vi "pixelfly_init.vi"(3 "error in (no error)":errorcluster, 4 "PixelFly Controls":T1={"Acquitsition Settings"={"Buffer number"=1, "Size (Bytes)"=150, "initialized array"=array2048x1280[2621440 elements], "X Bin"=1, "Y Bin"=0, "Board Handle"=0, "Picture parameters"={"ccdxsize"=0, "ccdy"=0, "pictx"=0, "picty"=0, "bitspixel"=12}, "Buffer Out"=[]}, "Initialization"={"Exposure mode"=1, "exp time"=150, "exp level"=1, "gain"=0, "boardid in"=0, "offset"=0, "V bin"=0, "H bin"=0, "trigger"=TRUE, "Bit depth"=0}} {"Initialization"."Bit depth" items=["8", "12"]; "Initialization"."H bin" items=["1", "2"]; "Initialization"."V bin" items=["1", "2"]; "Initialization"."boardid in" min=0 max=3 step=1; "Initialization"."gain" items=["Low (X1)", "High (X2)"]; "Initialization"."exp level" min=0 max=255 step=1; "Initialization"."exp time" min=1 max=10000; "Initialization"."Exposure mode" items=["Asynch shutter", "Double shot", "Video mode", "Auto exposure"]}) -> (0 "error out":errorcluster, 1 "PixelFly Status":T4 {"CCD temp" scale=0.0..100.0; "Board Parameters"."Vertical bin" items=["1", "2"]; "Board Parameters"."Horizontal bin" items=["1", "2"]}, 2 "PixelFly Controls Out":T1={"Acquitsition Settings"={"Buffer number"=1, "Size (Bytes)"=150, "initialized array"=array2048x1280[2621440 elements], "X Bin"=1, "Y Bin"=0, "Board Handle"=0, "Picture parameters"={"ccdxsize"=0, "ccdy"=0, "pictx"=0, "picty"=0, "bitspixel"=12}, "Buffer Out"=[]}, "Initialization"={"Exposure mode"=1, "exp time"=150, "exp level"=1, "gain"=0, "boardid in"=0, "offset"=0, "V bin"=0, "H bin"=0, "trigger"=TRUE, "Bit depth"=0}} {"Initialization"."Bit depth" items=["8", "12"]; "Initialization"."H bin" items=["1", "2"]; "Initialization"."V bin" items=["1", "2"]; "Initialization"."boardid in" min=0 max=3 step=1; "Initialization"."gain" items=["Low (X1)", "High (X2)"]; "Initialization"."exp level" min=0 max=255 step=1; "Initialization"."exp time" min=1 max=10000; "Initialization"."Exposure mode" items=["Asynch shutter", "Double shot", "Video mode", "Auto exposure"]})   [LabVIEW 2016]
doc: "Initializes the PixelFly camera and prepares it for 'pixelfly_acquire' to take images. Note that 'pixelfly_close' should be run when done imaging."
uses:
  Controls/PixelFly/PixelFly_Control.ctl
  Controls/PixelFly/Acquisition Settings.ctl
  Controls/PixelFly/Bit_Depth_Enum.ctl
  Controls/PixelFly/PixelFly Status Indicator.ctl
panel:
  # "Camera Controls"
  # "Camera Indicators"
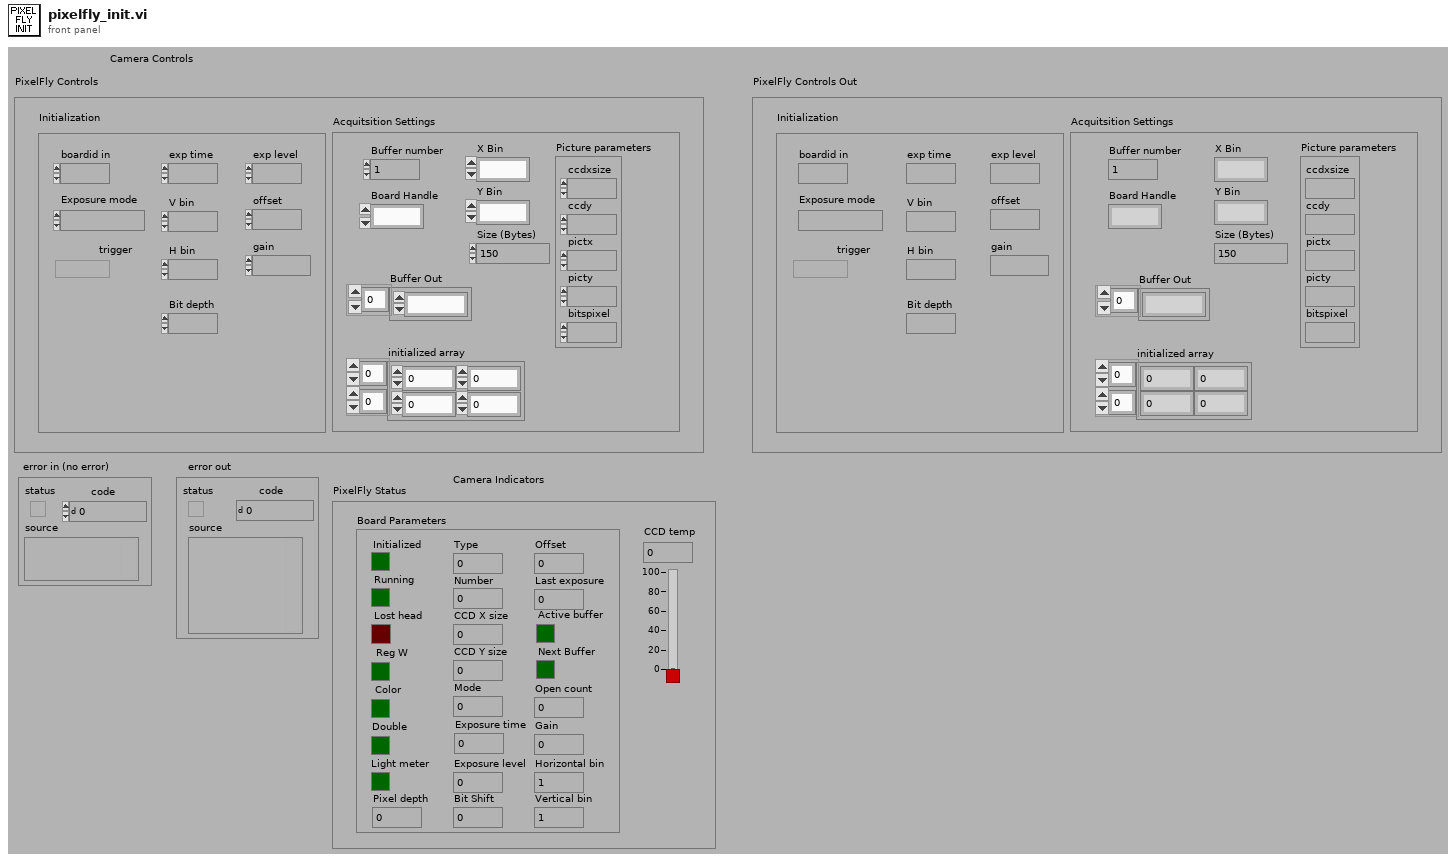
[diagram p1: front panel]
types:
  T1 = typedef "PixelFly_Control.ctl" = cluster{"Acquitsition Settings":T2, "Initialization":cluster{"Exposure mode":u16, "exp time":i32, "exp level":i32, "gain":i32, "boardid in":i32, "offset":i32, "V bin":i32, "H bin":i32, "trigger":bool, "Bit depth":T3}}
  T2 = typedef "Acquisition Settings.ctl" = cluster{"Buffer number":i32, "Size (Bytes)":i32, "initialized array":u16[][], "X Bin":i32, "Y Bin":i32, "Board Handle":u32, "Picture parameters":cluster{"ccdxsize":i32, "ccdy":i32, "pictx":i32, "picty":i32, "bitspixel":i32}, "Buffer Out":u16[]}
  T3 = typedef "Bit_Depth_Enum.ctl" = i32
  T4 = typedef "PixelFly Status Indicator.ctl" = cluster{"Board Parameters":cluster{"Type":u32, "Number":u32, "Initialized":bool, "Running":bool, "Lost head":bool, "CCD X size":u32, "CCD Y size":u32, "Mode":u32, "Exposure time":u32, "Exposure level":u32, "Horizontal bin":u32, "Vertical bin":u32, "Reg W":bool, "Gain":u32, "Pixel depth":i32, "Bit Shift":u32, "Offset":u32, "Last exposure":u32, "Double ":bool, "Light meter":bool, "Color":bool, "Open count":u32, "Active buffer":bool, "Next Buffer":bool}, "CCD temp":i32}
  T5 = cluster{"Type":u32, "Number":u32, "Initialized":bool, "Running":bool, "Lost head":bool, "CCD X size":u32, "CCD Y size":u32, "Mode":u32, "Exposure time":u32, "Exposure level":u32, "Horizontal bin":u32, "Vertical bin":u32, "Reg W":bool, "Gain":u32, "Pixel depth":i32, "Bit Shift":u32, "Offset":u32, "Last exposure":u32, "Double ":bool, "Light meter":bool, "Color":bool, "Open count":u32, "Active buffer":bool, "Next Buffer":bool}
  T6 = cluster{"ccdxsize":i32, "ccdy":i32, "pictx":i32, "picty":i32, "bitspixel":i32}
  T7 = cluster{"Board Parameters":cluster{"Type":u32, "Number":u32, "Initialized":bool, "Running":bool, "Lost head":bool, "CCD X size":u32, "CCD Y size":u32, "Mode":u32, "Exposure time":u32, "Exposure level":u32, "Horizontal bin":u32, "Vertical bin":u32, "Reg W":bool, "Gain":u32, "Pixel depth":i32, "Bit Shift":u32, "Offset":u32, "Last exposure":u32, "Double ":bool, "Light meter":bool, "Color":bool, "Open count":u32, "Active buffer":bool, "Next Buffer":bool}, "CCD temp":i32}
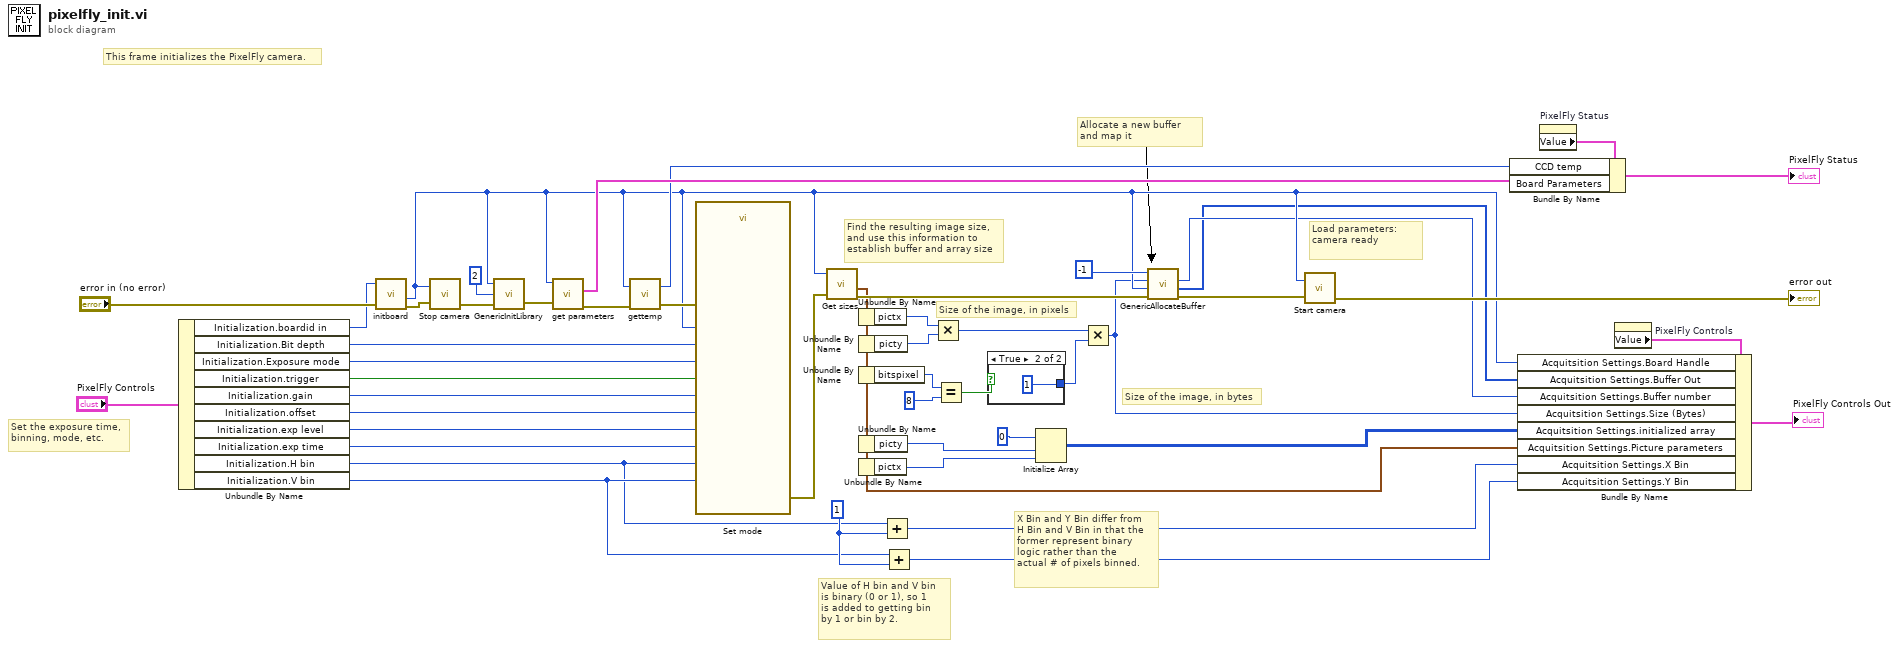
[diagram p0: block diagram]
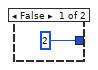
[diagram p2: hidden frame]
diagram:
  w35 = 1
  # "Value of H bin and V bin\nis binary (0 or 1), so 1\nis added to getting bin\nby 1 or bin by 2."
  # "X Bin and Y Bin differ from\nH Bin and V Bin in that the\nformer represent binary\nlogic rather than the\nactual # of pixels binned."
  # "Load parameters: camera ready"
  # "Allocate a new buffer and map it"
  # "Find the resulting image size, and use this information to establish buffer and array size"
  # "Size of the image, in pixels"
  # "Size of the image, in bytes"
  # "This frame initializes the PixelFly camera."
  # "Set the exposure time, binning, mode, etc."
  n1 = Unbundle By Name("PixelFly Controls") -> ("Initialization.boardid in"=w32:i32, "Initialization.Bit depth"=w31:T3, "Initialization.Exposure mode"=w30:u16, "Initialization.trigger"=w29:bool, "Initialization.gain"=w28:i32, "Initialization.offset"=w27:i32, "Initialization.exp level"=w26:i32, "Initialization.exp time"=w25:i32, "Initialization.H bin"=w23:i32, "Initialization.V bin"=w24:i32)
  n2 = call "initboard.vi"("boardid in"=w32, "error in (no error)"="error in (no error)") -> ("hOut"=w9:u32, "error out"=w14:errorcluster)  [unwired: 1 in, 2 out]
  n3 = call "Stop camera.vi"("Handle in"=w9, "error in (no error)"=w14) -> ("error out"=w13:errorcluster)  [unwired: 2 out]
  n4 = call "GenericInitLibrary.vi"("error in (no error)"=w13, "Interface Type"=u32 2, "hIn"=w9) -> ("error out"=w16:errorcluster)  [unwired: 1 in]
  n5 = call "get parameters.vi"("error in (no error)"=w16, "Handle in"=w9) -> ("error out"=w34:errorcluster, "Board Parameters"=w19:T5)  [unwired: 2 in, 2 out]
  n6 = call "gettemp.vi"("Handle in"=w9, "error in (no error)"=w34) -> ("ccdtemp"=w18:i32, "error out"=w33:errorcluster)  [unwired: 1 out]
  n7 = call "Set mode.vi"("Exposure mode"=w30, "Handle in"=w9, "offset"=w27, "bits/pixel"=w31, "trigger"=w29, "exp level"=w26, "H bin"=w23, "V bin"=w24, "exp time"=w25, "gain"=w28, "error in (no error)"=w33) -> ("error out"=w46:errorcluster)  [unwired: 4 in]
  n8 = call "Get sizes.vi"("Handle in"=w9, "error in (no error)"=w46) -> ("Picture parameters"=w2:T6, "error out"=w12:errorcluster)  [unwired: 1 in, 2 out]
  n9 = Unbundle By Name(w2) -> ("pictx"=w45:i32)
  n10 = Unbundle By Name(w2) -> ("picty"=w44:i32)
  n11 = Unbundle By Name(w2) -> ("bitspixel"=w43:i32)
  n12 = Unbundle By Name(w2) -> ("picty"=w37:i32)
  n13 = Unbundle By Name(w2) -> ("pictx"=w36:i32)
  n14 = Add(x=w23, y=w35) -> (x+y=w3:i32)
  n15 = Add(x=w24, y=w35) -> (x+y=w22:i32)
  n16 = Multiply(x=w45, y=w44) -> (x*y=w40:i32)
  n17 = Equal?(x=w43, y=8) -> (x = y?=w41:bool)
  n18 = case shown="True" w41 {
    tunnel: [2 1] -> w39
    frame False {
    }
    frame True {
    }
  }
  n19 = Initialize Array(u16 0 ("16 bit integers"), w37, w36) -> (w21:u16[][])
  n20 = Multiply(x=w40, y=w39) -> (x*y=w6:i32)
  n21 = call "GenericAllocateBuffer.vi"("BufNr"=i16 -1, "Size"=w6, "ph"=w9, "error in (no error)"=w12) -> ("BufNrOut"=w8:i16, "BufOut"=w7:u16[], "error out"=w11:errorcluster)  [unwired: 2 out]
  n22 = call "Start camera.vi"("Handle in"=w9, "error in (no error)"=w11) -> ("error out"=→"error out":errorcluster)  [unwired: 2 out]
  n23 = property on="PixelFly Status" class="Clust (strict)"() -> ("Value"=w20:T7)  [unwired: 2 in, 2 out]
  n24 = Bundle By Name(cluster=w20, "CCD temp"=w18, "Board Parameters"=w19) -> (→"PixelFly Status":T7)
  n25 = property on="PixelFly Controls" class="Clust (strict)"() -> ("Value"=w4:T1)  [unwired: 2 in, 2 out]
  n26 = Bundle By Name(cluster=w4, "Acquitsition Settings.Board Handle"=w9, "Acquitsition Settings.Buffer Out"=w7, "Acquitsition Settings.Buffer number"=w8, "Acquitsition Settings.Size (Bytes)"=w6, "Acquitsition Settings.initialized array"=w21, "Acquitsition Settings.Picture parameters"=w2, "Acquitsition Settings.X Bin"=w3, "Acquitsition Settings.Y Bin"=w22) -> (→"PixelFly Controls Out":T1)
